vi "clear_usb_buffer.vi"(0 "reference":i32, 5 "error in (no error)":errorcluster) -> (19 "error out":errorcluster)   [LabVIEW 2012]
doc: "Clears the buffer on the PC as well as the USB controller. \n\nImplementss the USB Communication API function \"fnPerformaxComFlush\".\n\nProduced By:\n\nChristopher Lemieux\nKod Integrations, LLC\n4835 Marianne Drive\nMount Airy, MD 21771\nhttp://www.kodintegrations.com\nemail: clemieux@kodintegrations.com\nphone: (240) 687-1288"
uses:
  support/controls/errors_actions.ctl
  PerformaxCom.dll
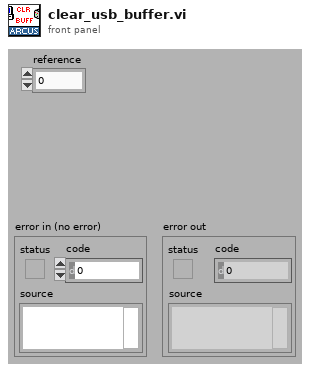
[diagram p1: front panel]
types:
  T1 = typedef "errors_actions.ctl" = enum16{"clearBuff", "closeRef", "noDeviceInfo", "noDevices", "openRef", "sendReceive", "setTimeouts", "unknown"}
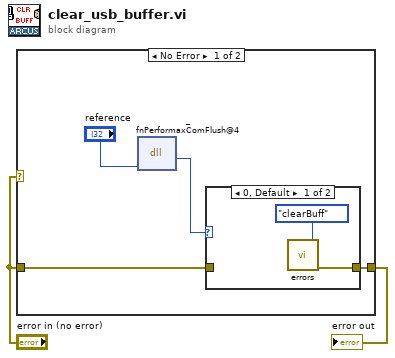
[diagram p0: block diagram]
diagram:
  n1 = case shown="No Error" "error in (no error)" {
    tunnel: "error in (no error)" -> [w6 w10]
    tunnel: [w5 w10] -> w1
    frame No Error {
      n2 = dll-call lib="PerformaxCom.dll" fn="_fnPerformaxComFlush@4"("reference"="reference") -> ("success"=w4:i32)  [unwired: 4 in, 2 out]
      n3 = case shown="0, Default" w4 {
        tunnel: [w7 w9] -> w5
        tunnel: w6 -> [_ w9]
        frame 0, Default {
          n4 = call "errors.vi"("errors"=errors_actions."clearBuff") -> ("error out"=w7:errorcluster)  [unwired: 14 in]
        }
        frame 1 {
        }
      }
    }
    frame Error {
    }
  }
  "error out" <- w1
